vi "Lambda filter.vi"(10 "Lambda in":dbl) -> (2 "Labmda out":dbl)   [LabVIEW 2011]
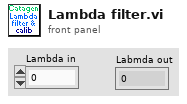
[diagram p1: front panel]
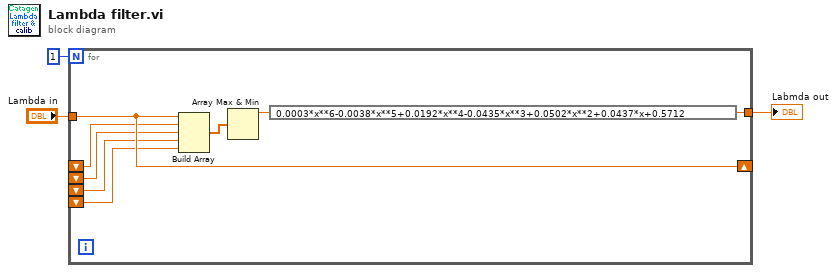
[diagram p0: block diagram]
diagram:
  n1 = for {
    N: 1 -> [_]
    tunnel: [w11] -> w3
    tunnel: "Lambda in" -> [w8]
    shift-right: [w8] -> _
    shift-left: _ -> [w7]
    shift-left: _ -> [w6]
    shift-left: _ -> [w5]
    shift-left: _ -> [w4]
    n2 = Build Array(w8, w7, w6, w5, w4) -> (w10:dbl[])
    n3 = Array Max & Min(array=w10) -> (max value=w9:dbl)  [unwired: 3 out]
    n4 = expression code="0.0003*x**6-0.0038*x**5+0.0192*x**4-0.0435*x**3+0.0502*x**2+0.0437*x+0.5712"(w9) -> (w11:dbl)
  }
  "Labmda out" <- w3
